vi "Extract all ROI info.vi"() -> (1 "Zero-based index of the Z-plane the indexed ROI belongs to":i32[](array[numeric]), 3 "[ROI info]":T1[](array[typedef]) {"ROI group ID" format="%#_6f"; "Laser Power (%)" format="%#_6f"; "Zoom" format="%#_6f"; "Frame Size" format="%#_6f"; "Number of lines" format="%#_6f"; "Composite ID" format="%#_6f"; "Angle (deg)" format="%#_6f"; "ROI Time (ns)" format="%#_6f"; "ROI ID" format="%#_6f"; "Pixels in ROI" format="%#_6f"; "ROI index" format="%#_6f"; "Z stop" format="%#_6f"; "Y stop" format="%#_6f"; "X stop" format="%#_6f"; "Z start" format="%#_6f"; "X start" format="%#_6f"; "Y start" format="%#_6f"})   [LabVIEW 2017]
uses:
  Typedefs/ROI parameters data type.ctl
  Typedefs/Get-Set-Clear Control.ctl
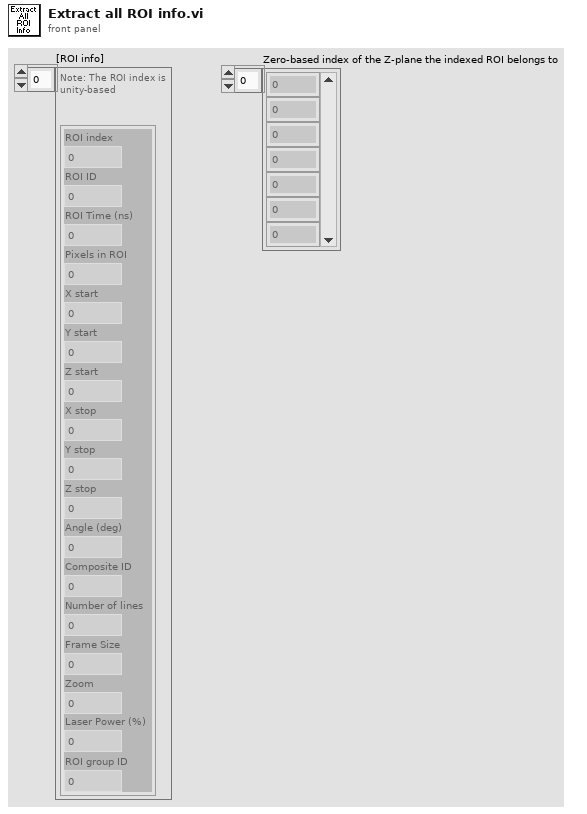
[diagram p1: front panel]
types:
  T1 = typedef "ROI parameters data type.ctl" = cluster{"ROI index":dbl, "ROI ID":dbl, "ROI Time (ns)":dbl, "Pixels in ROI":dbl, "X start":dbl, "Y start":dbl, "Z start":dbl, "X stop":dbl, "Y stop":dbl, "Z stop":dbl, "Angle (deg)":dbl, "Composite ID":dbl, "Number of lines":dbl, "Frame Size":dbl, "Zoom":dbl, "Laser Power (%)":dbl, "ROI group ID":dbl}
  T2 = typedef "Get-Set-Clear Control.ctl" = enum16{"Get", "Set", "Clear"}
  T3 = typedef "Functional Parameters Cluster.ctl" = cluster{"ROI data":dbl[][], "ROI format version":i32, "Norm ROI data":dbl[][], "Norm. ROI format version":i32, "Z norm":dbl[], "Z norm format version":i32}
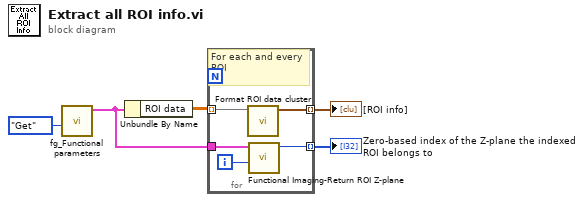
[diagram p0: block diagram]
diagram:
  n1 = call "fg_Functional parameters.vi"("Function"=Get-Set-Clear_Control."Get") -> ("Functional Parameters"=w3:T3)  [unwired: 7 in, 3 out]
  n2 = Unbundle By Name(w3) -> ("ROI data"=w1:dbl[][])
  n3 = for {
    tunnel: [w10] -> w5 mode=indexing
    tunnel: w1 -> [w9] mode=indexing
    tunnel: w3 -> [w8]
    tunnel: [w6] -> w4 mode=indexing
    i -> [w7]
    # "For each and every ROI"
    n4 = call "Format ROI data cluster.vi"("Single ROI info"=w9) -> ("X-Y-Z coordinates"=w10:T1)  [unwired: 10 in]
    n5 = call "Functional Imaging-Return ROI Z-plane.vi"("ROI index (zero based)"=w7, "Functional Parameters"=w8) -> ("Zero-based index of the Z-plane the indexed ROI belongs to"=w6:i32)  [unwired: 9 in]
  }
  "[ROI info]" <- w5
  "Zero-based index of the Z-plane the indexed ROI belongs to" <- w4
